vi "TL hindbrain THINK.vi"(2 "error in":errorcluster) -> (0 "error out":errorcluster)   [LabVIEW 2014]
doc: "This vi is the THINK portion of the Hindbrain...at present it has not function and is a place holder for later development."
panel:
  # "AT PRESENT THIS IS JUST A PLACE HOLDER"
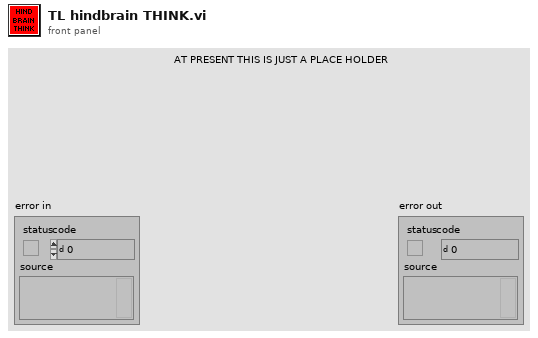
[diagram p1: front panel]
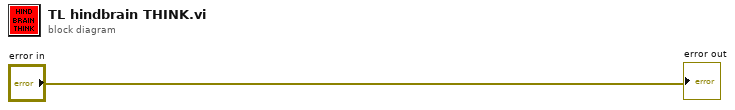
[diagram p0: block diagram]
diagram:
  "error out" <- "error in"
